vi "AddHintCallback.vi"(8 "No Error":errorcluster, 9 "Userdata [void *]":i64, 10 "Callback [SDL_HintCallback]":i64, 11 "Hint Name":T1) -> (0 "error out":errorcluster)   [LabVIEW 2024, in "SDL3.lvlib" / "Hints.lvlib"]
doc: "<B>Summary</B>\nAdd a function to watch a particular hint.\n\n<B>Remarks</B>\nThe callback function is called during this function, to provide it an initial value, and again each time the hint's value changes."
uses:
  Hints.lvlib
  Lib/SDL3.dll
  HintName--combobox.ctl
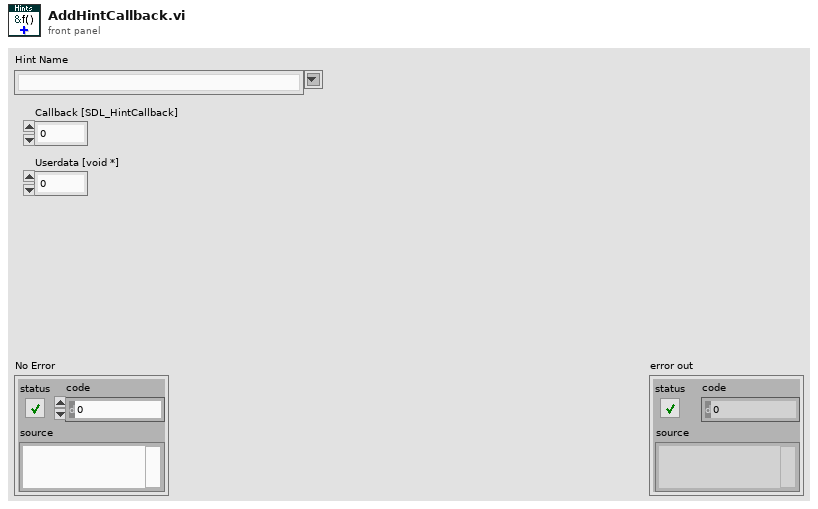
[diagram p1: front panel]
types:
  T1 = typedef "SDL3.lvlib/Hints.lvlib/HintName--combobox.ctl" = string
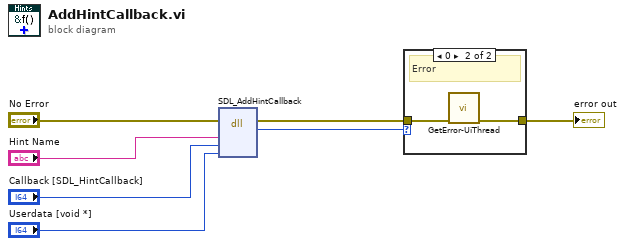
[diagram p0: block diagram]
diagram:
  n1 = dll-call lib="C:/Users/Thomas/Documents/Projects/LV-SDL3/Sources/SDL3/Lib/SDL3.*" fn="SDL_AddHintCallback"(error in="No Error", "name"="Hint Name", "callback"="Callback [SDL_HintCallback]", "userdata"="Userdata [void *]") -> (error out=w5:errorcluster, "return type"=w3:i32)  [unwired: 5 in, 1 out]
  n2 = case shown="0" w3 {
    tunnel: w5 -> [w8 w10]
    tunnel: [w8 w9] -> w4
    frame Default {
      # "Ok"
    }
    frame 0 {
      # "Error"
      n3 = call "GetError-UiThread.vi"("No Error"=w10) -> ("error out"=w9:errorcluster)  [unwired: 10 in]
    }
  }
  "error out" <- w4
